vi "PH_Beckhoff_Application.read DB.vi"(2 "error in":errorcluster, 3 "Instance Name":string) -> (0 "error out":errorcluster, 1 "Beckhoff Type":T1)   [LabVIEW 2014, in "PH_Beckhoff_Application.lvlib"]
doc: "This VI reads information from the database and writes it to own attributes."
uses:
  PH_Beckhoff_Application.lvlib
  PH_Beckhoff_Application.Beckhoff Type.ctl
  PH_Basics/PH_Common/PH_Common.lvlib
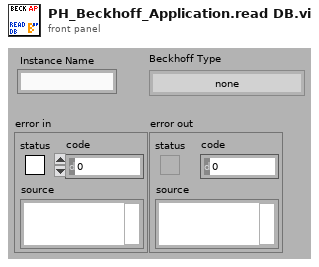
[diagram p1: front panel]
types:
  T1 = typedef "PH_Beckhoff_Application.lvlib/PH_Beckhoff_Application.Beckhoff Type.ctl" = enum16{"none", "PILS internal", "PILS external", "Timing", "MA 01"}
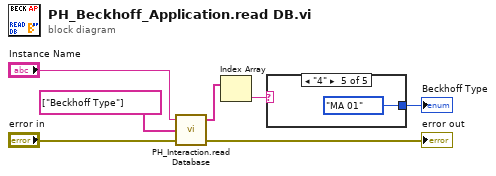
[diagram p0: block diagram]
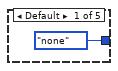
[diagram p2: hidden frame]
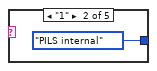
[diagram p3: hidden frame]
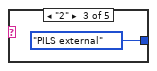
[diagram p4: hidden frame]
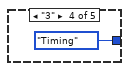
[diagram p5: hidden frame]
diagram:
  n1 = call "PH_Interaction.read Database.vi"("error in (no error)"="error in", "Strings to search for"=string[] ["Beckhoff Type"] ("Strings to search for in"), "DB Entry to read"="Instance Name") -> ("error out"=→"error out":errorcluster, "Values"=w4:string[])  [unwired: 1 in]
  n2 = Index Array(array=w4) -> (element=w3:string)  [unwired: 1 in]
  n3 = case shown="\"4\"" w3 {
    tunnel: [PH_Beckhoff_Application.Beckhoff_Type."none" ("Beckhoff Type") PH_Beckhoff_Application.Beckhoff_Type."PILS internal" ("Beckhoff Type") PH_Beckhoff_Application.Beckhoff_Type."PILS external" ("Beckhoff Type") PH_Beckhoff_Application.Beckhoff_Type."Timing" ("Beckhoff Type") PH_Beckhoff_Application.Beckhoff_Type."MA 01" ("Beckhoff Type")] -> w5
    frame Default {
    }
    frame "1" {
    }
    frame "2" {
    }
    frame "3" {
    }
    frame "4" {
    }
  }
  "Beckhoff Type" <- w5
